vi "RGseriesSerialTest_dual.vi"() -> ()   [LabVIEW 2009]
uses:
  <vilib>/Instr/_visa.llb/VISA Configure Serial Port (Instr).vi
panel:
  out "return count 8":u32
  out "return count 7":u32
  out "return count 6":u32
  out "return count 5":u32
  out "ICN MES A":dbl
  out "VCN MES V":dbl
  out "return count 4":u32
  out "return count 3":u32
  out "return count 2":u32
  out "return count":u32
  out "VCN MES":string
  in  "VISA resource name":refnum<visa-resource-name>
  in  "timeout (10sec)":u32=10000
  out "ICN MES":string
  out "VCN_REQ_COM":string
  out "ICN_REQ_COM":string
  in  "VCN_REQ":dbl(knob) scale=0.0..15.0
  in  "ICN_REQ":dbl(knob) scale=0.0..3.0
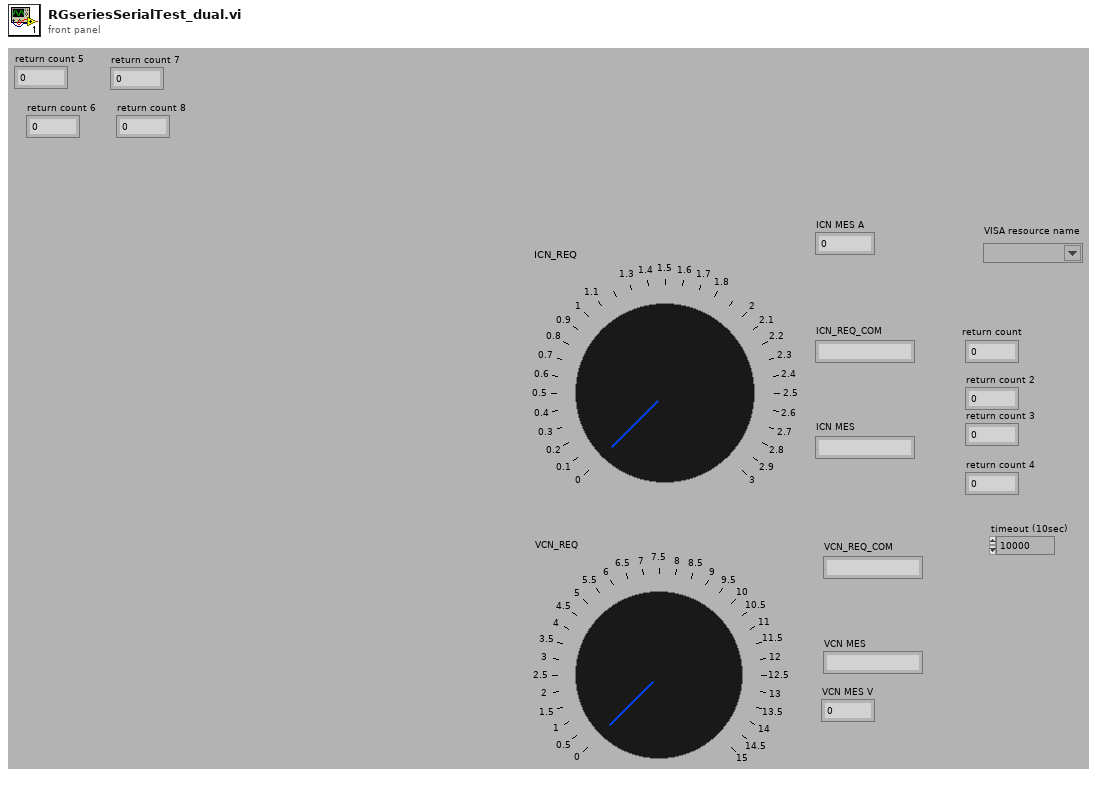
[diagram p1: front panel]
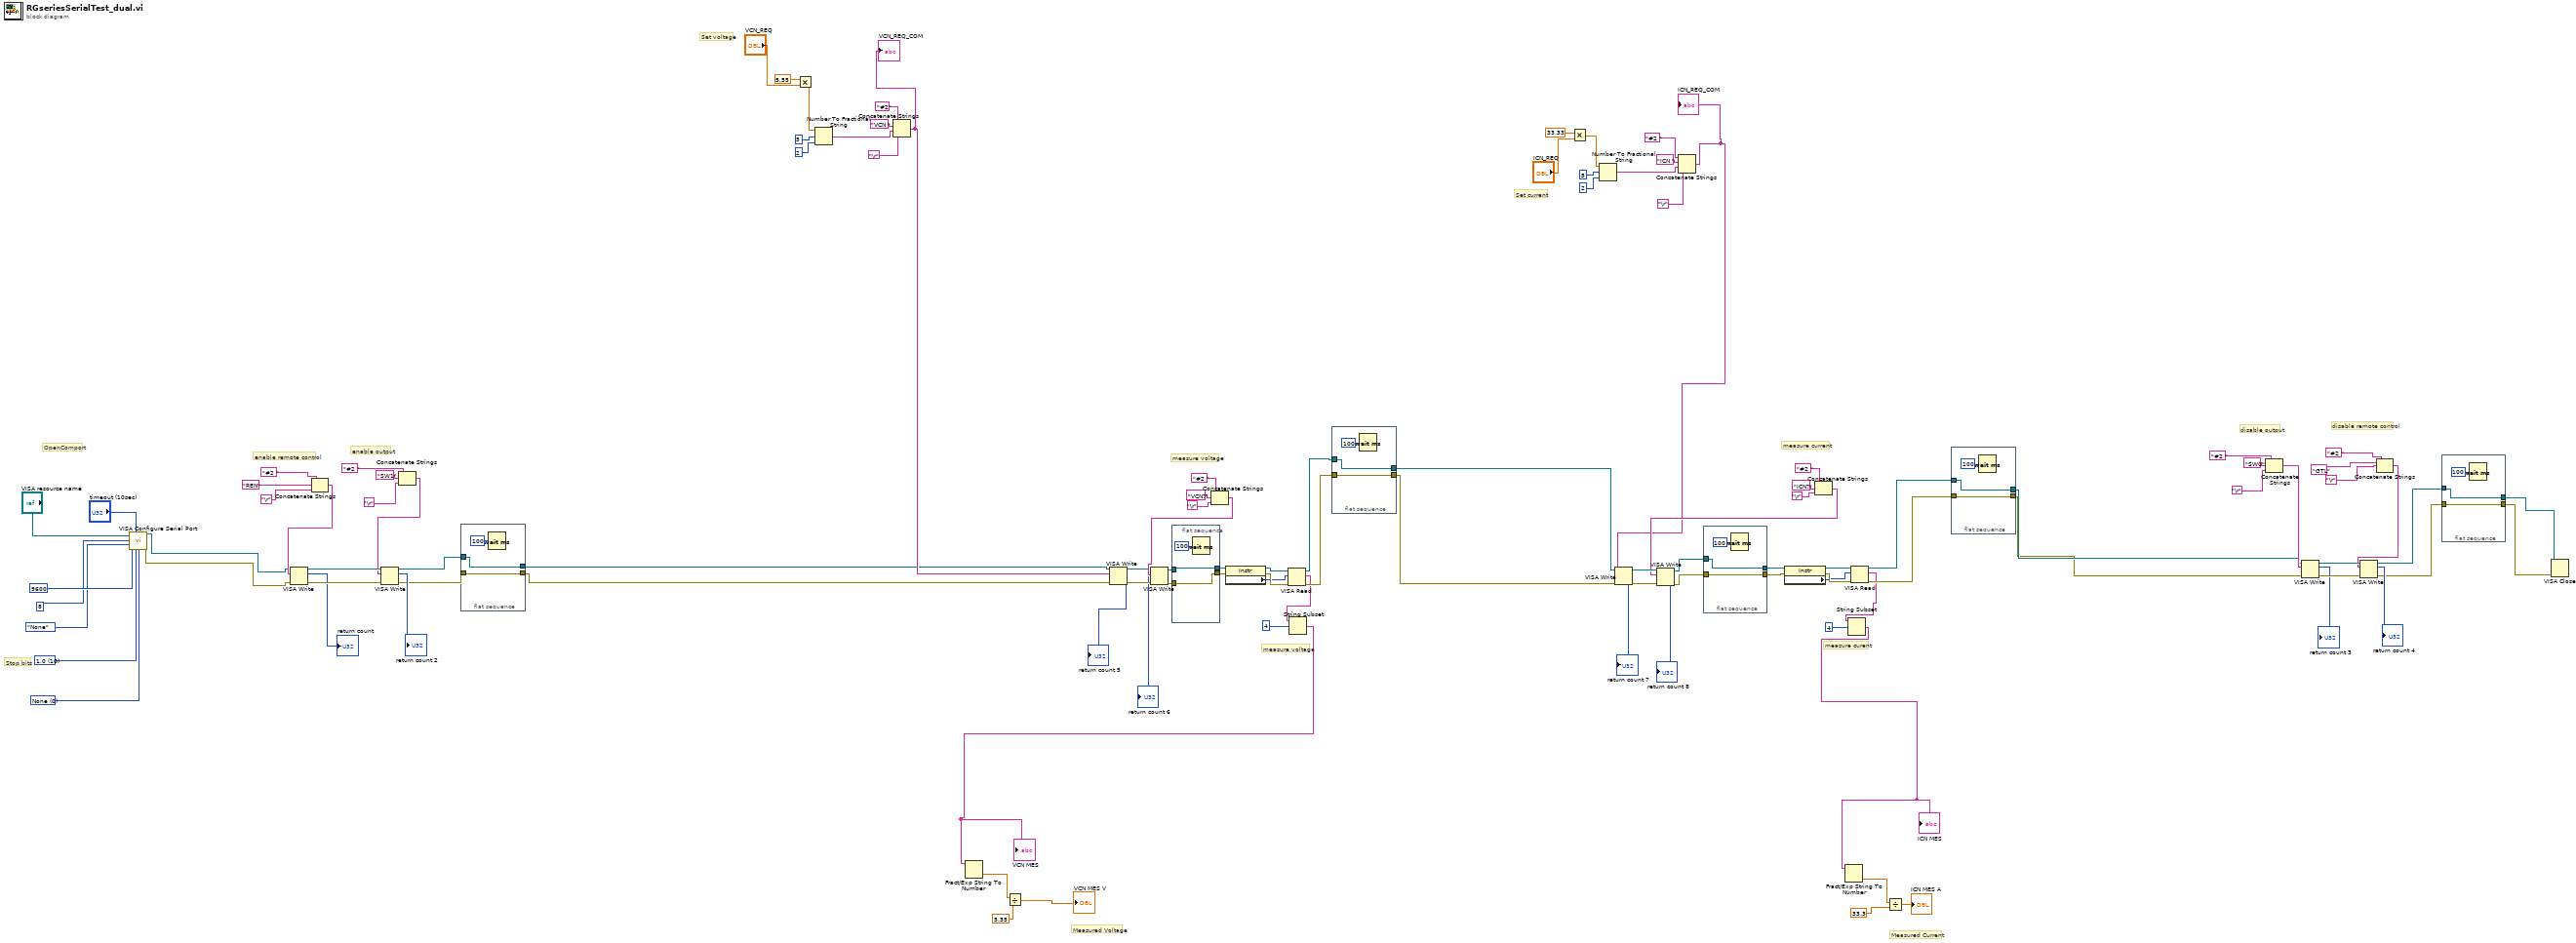
[diagram p0: block diagram]
diagram:
  w95 = u16 0 items=["None", "XON/XOFF", "RTS/CTS", "XON/XOFF & RTS/CTS", "DTR/DSR", "XON/XOFF & DTR/DSR"] ("flow control (0:none)")
  w96 = u16 10 items=["1.0"=10, "1.5"=15, "2.0"=20] ("stop bits (10: 1 bit)")
  # "measure current"
  # "measure voltage"
  # "measure voltage"
  # "measure curent"
  # "OpenComport"
  # "Measured Voltage"
  # "Measured Current"
  # "Set current"
  # "Set voltage"
  # "Stop bits"
  # "enable remote control"
  # "enable output"
  # "disable remote control"
  # "disable output"
  n1 = call-poly "VISA Configure Serial Port"("VISA resource name"="VISA resource name", "timeout (10sec)"="timeout (10sec)", "baud rate (9600)"=u32 9600, "data bits (8)"=u16 8, "parity (0:none)"=enum16{"None", "Odd", "Even", "Mark", "Space"}."None", "stop bits (10: 1 bit)"=w96, "flow control (0:none)"=w95) -> ("VISA resource name out"=w86:refnum<visa-resource-name>, "error out"=w85:errorcluster)  [unwired: 7 in]
  n2 = Concatenate Strings("#2 " ("initial string"), "REN" ("string"), "\r") -> (w92:string)
  n3 = VISA Write(VISA resource name=w86, write buffer=w92, error in (no error)=w85) -> (VISA resource name out=w94:refnum<visa-resource-name>, return count=→"return count":u32, error out=w93:errorcluster)
  n4 = Concatenate Strings("#2 " ("format string"), "SW1" ("initial string"), "\r" ("input 1")) -> (w91:string)
  n5 = VISA Write(VISA resource name=w94, write buffer=w91, error in (no error)=w93) -> (VISA resource name out=w55:refnum<visa-resource-name>, return count=→"return count 2":u32, error out=w56:errorcluster)
  n6 = flat-sequence {
    tunnel: w55 -> [w112]
    tunnel: w56 -> [w113]
    tunnel: [w113] -> w3
    tunnel: [w112] -> w4
    frame #0 {
      n7 = Wait (ms)(milliseconds to wait=u32 100) -> ()  [unwired: 1 out]
    }
  }
  n8 = Multiply(x=5.55, y="VCN_REQ") -> (x*y=w75:dbl)
  n9 = Number To Fractional String(number=w75, width (-)=i16 5, precision (6)=i16 2) -> (F-format string=w77:string)  [unwired: 1 in]
  n10 = Concatenate Strings("#2" ("format string"), "VCN " ("initial string"), w77, "\r") -> (w8:string)
  "VCN_REQ_COM" <- w8
  n11 = VISA Write(VISA resource name=w4, write buffer=w8, error in (no error)=w3) -> (VISA resource name out=w42:refnum<visa-resource-name>, return count=→"return count 5":u32, error out=w41:errorcluster)
  n12 = flat-sequence {
    tunnel: w24 -> [w117]
    tunnel: [w117] -> w23
    tunnel: w22 -> [w116]
    tunnel: [w116] -> w21
    frame #0 {
      n13 = Wait (ms)(milliseconds to wait=u32 100) -> ()  [unwired: 1 out]
    }
  }
  n14 = Concatenate Strings("#2 " ("format string"), "VCN?" ("initial string"), "\r" ("input 1")) -> (w43:string)
  n15 = VISA Write(VISA resource name=w42, write buffer=w43, error in (no error)=w41) -> (VISA resource name out=w24:refnum<visa-resource-name>, return count=→"return count 6":u32, error out=w22:errorcluster)
  n16 = property class="Instr"(reference=w23, error in=w21) -> (reference out=w30:refnum<visa-resource-name>, error out=w29:errorcluster, "Serial Settings:Number of Bytes at Serial Port"=w28:u32)
  n17 = VISA Read(VISA resource name=w30, byte count=w28, error in (no error)=w29) -> (VISA resource name out=w16:refnum<visa-resource-name>, read buffer=w9:string, error out=w15:errorcluster)  [unwired: 1 out]
  n18 = String Subset(string=w9, offset (0)=4) -> (substring=w6:string)  [unwired: 1 in]
  "VCN MES" <- w6
  n19 = Fract/Exp String To Number(string=w6) -> (number=w52:dbl)  [unwired: 3 in, 1 out]
  n20 = Divide(x=w52, y=5.55 ("x")) -> (x/y=→"VCN MES V":dbl)
  n21 = flat-sequence {
    tunnel: w16 -> [w119]
    tunnel: w15 -> [w118]
    tunnel: [w119] -> w13
    tunnel: [w118] -> w14
    frame #0 {
      n22 = Wait (ms)(milliseconds to wait=u32 100) -> ()  [unwired: 1 out]
    }
  }
  n23 = Multiply(x=33.33, y="ICN_REQ") -> (x*y=w65:dbl)
  n24 = Number To Fractional String(number=w65, width (-)=i16 5, precision (6)=i16 2) -> (F-format string=w68:string)  [unwired: 1 in]
  n25 = Concatenate Strings("#2 " ("initial string"), "ICN " ("initial string"), w68, "\r") -> (w7:string)
  "ICN_REQ_COM" <- w7
  n26 = VISA Write(VISA resource name=w13, write buffer=w7, error in (no error)=w14) -> (VISA resource name out=w38:refnum<visa-resource-name>, return count=→"return count 7":u32, error out=w39:errorcluster)
  n27 = flat-sequence {
    tunnel: w20 -> [w122]
    tunnel: w19 -> [w121]
    tunnel: [w122] -> w18
    tunnel: [w121] -> w17
    frame #0 {
      n28 = Wait (ms)(milliseconds to wait=u32 100) -> ()  [unwired: 1 out]
    }
  }
  n29 = property class="Instr"(reference=w18, error in=w17) -> (reference out=w27:refnum<visa-resource-name>, error out=w26:errorcluster, "Serial Settings:Number of Bytes at Serial Port"=w25:u32)
  n30 = Concatenate Strings("#2 " ("format string"), "ICN?" ("initial string"), "\r" ("input 1")) -> (w36:string)
  n31 = VISA Write(VISA resource name=w38, write buffer=w36, error in (no error)=w39) -> (VISA resource name out=w20:refnum<visa-resource-name>, return count=→"return count 8":u32, error out=w19:errorcluster)
  n32 = VISA Read(VISA resource name=w27, byte count=w25, error in (no error)=w26) -> (VISA resource name out=w12:refnum<visa-resource-name>, read buffer=w10:string, error out=w11:errorcluster)  [unwired: 1 out]
  n33 = String Subset(string=w10, offset (0)=4) -> (substring=w5:string)  [unwired: 1 in]
  "ICN MES" <- w5
  n34 = Fract/Exp String To Number(string=w5) -> (number=w49:dbl)  [unwired: 3 in, 1 out]
  n35 = Divide(x=w49, y=33.3 ("x")) -> (x/y=→"ICN MES A":dbl)
  n36 = flat-sequence {
    tunnel: w12 -> [w124]
    tunnel: w11 -> [w125]
    tunnel: [w125] -> w1
    tunnel: [w124] -> w2
    frame #0 {
      n37 = Wait (ms)(milliseconds to wait=u32 100) -> ()  [unwired: 1 out]
    }
  }
  n38 = Concatenate Strings("#2 " ("format string"), "SW0" ("initial string"), "\r" ("input 1")) -> (w87:string)
  n39 = VISA Write(VISA resource name=w2, write buffer=w87, error in (no error)=w1) -> (VISA resource name out=w90:refnum<visa-resource-name>, return count=→"return count 3":u32, error out=w89:errorcluster)
  n40 = Concatenate Strings("#2 " ("initial string"), "\r", "GTL" ("input 1")) -> (w88:string)
  n41 = VISA Write(VISA resource name=w90, write buffer=w88, error in (no error)=w89) -> (VISA resource name out=w59:refnum<visa-resource-name>, return count=→"return count 4":u32, error out=w60:errorcluster)
  n42 = flat-sequence {
    tunnel: w59 -> [w128]
    tunnel: w60 -> [w127]
    tunnel: [w128] -> w58
    tunnel: [w127] -> w57
    frame #0 {
      n43 = Wait (ms)(milliseconds to wait=u32 100) -> ()  [unwired: 1 out]
    }
  }
  n44 = VISA Close(VISA resource name=w58, error in (no error)=w57) -> ()  [unwired: 1 out]
